vi "Execute.vi"(8 "error in (no error)":errorcluster, 9 "Workspace":T1, 10 "Cluster":T2={"I-O.lvclass"=refnum, "Gantry"=refnum, "Dispenser"="COM1"}, 11 "Pick and Place in":refnum<class "Pick and Place.lvclass">) -> (0 "error out":errorcluster, 2 "Control Out":T2={"I-O.lvclass"=refnum, "Gantry"=refnum, "Dispenser"="COM1"}, 3 "Pick and Place out":refnum<class "Pick and Place.lvclass">)   [LabVIEW 2021, in "Pick and Place.lvclass"]
uses:
  Pick and Place.lvclass
  Controller/Controllers.ctl
  Controller/I-O/I-O.lvclass
  C:/Program Files (x86)/Aerotech/A3200/LabVIEW/2010/Bin/Aerotech.A3200.dll
  Program Files (x86)/Aerotech/A3200/LabVIEW/2010/Bin/Aerotech.A3200.dll
  Workspace/Workspace.ctl
  Pick and Place Type.ctl
  Pick and Place.lvclass/Pick and Place.ctl
  4c518ff3-1de9-431e-b450-1fb7357d944a.vi
  Drivers/Aerotech A3200/Parameters/GetAxisParameterDouble.vi
  Controller/Motion/Motion.lvclass
  Drivers/Aerotech A3200/Aerotech.lvlib
  Controller/Motion/A3200/A3200.lvclass
  Controller/Controller.lvclass
  Workspace/Fixture.lvclass
panel:
  in  "Deactivate curtain?":bool
  out "Seconary Pickup time 2":timestamp
  out "Seconary Pickup time 1":timestamp
  out "milliseconds to wait":u32
  out "XYZTheta Out":dbl[](array[numeric])
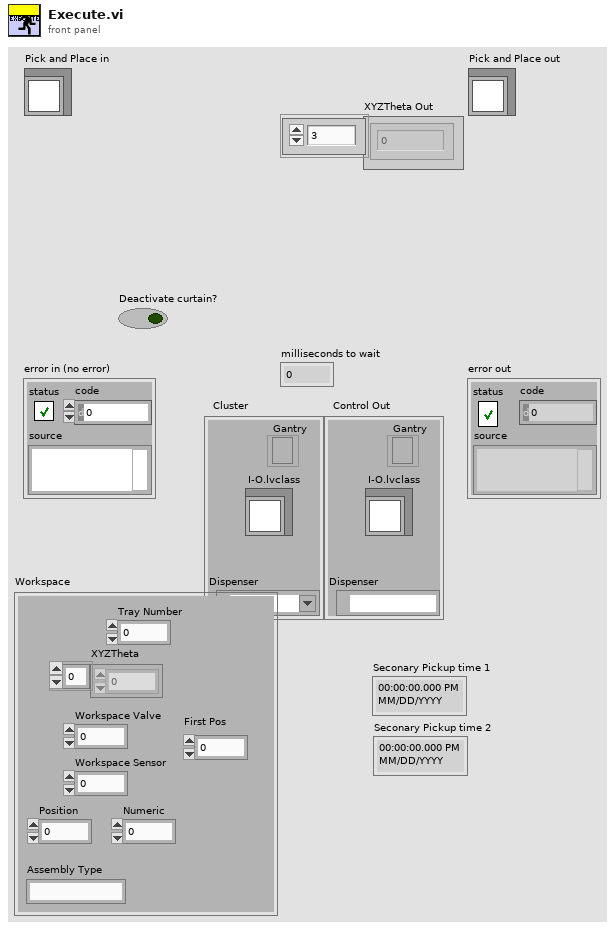
[diagram p1: front panel]
types:
  T1 = typedef "Fixture.lvclass/Workspace.ctl" = cluster{"XYZTheta":dbl[], "Workspace Valve":i32, "Workspace Sensor":i32, "Tray Number":i32, "Position":i32, "Assembly Type":string, "Numeric":dbl, "First Pos":i32}
  T2 = typedef "Controller.lvclass/Controllers.ctl" = cluster{"I-O.lvclass":refnum<class "I-O.lvclass">, "Gantry":refnum<k24>, "Dispenser":refnum<visa-resource-name>}
  T3 = typedef "Pick and Place.lvclass/Pick and Place Type.ctl" = enum16{"Primary Pick Up", "Secondary Pick Up", "Put Down All", "Pick Up All", "Put Down Secondary"}
  T4 = typedef "I-O.lvclass/Pin Map.ctl" = cluster{"Region Valves":i32[], "Extra Valves":dbl[][][], "Tool Primary Valve":i32, "Tool Secondary Valve":i32, "Region Sensors":i32[], "Extra Sensors":dbl[][][], "Tool Primary Sensor":dbl, "Tool Secondary Sensor":dbl, "Compression Sensor":dbl, "5V":i32, "Dispenser Sensor":dbl, "Light Curtain":i32}
  T5 = cluster{"Status":bool, "Error Code":i32, "Source":string}
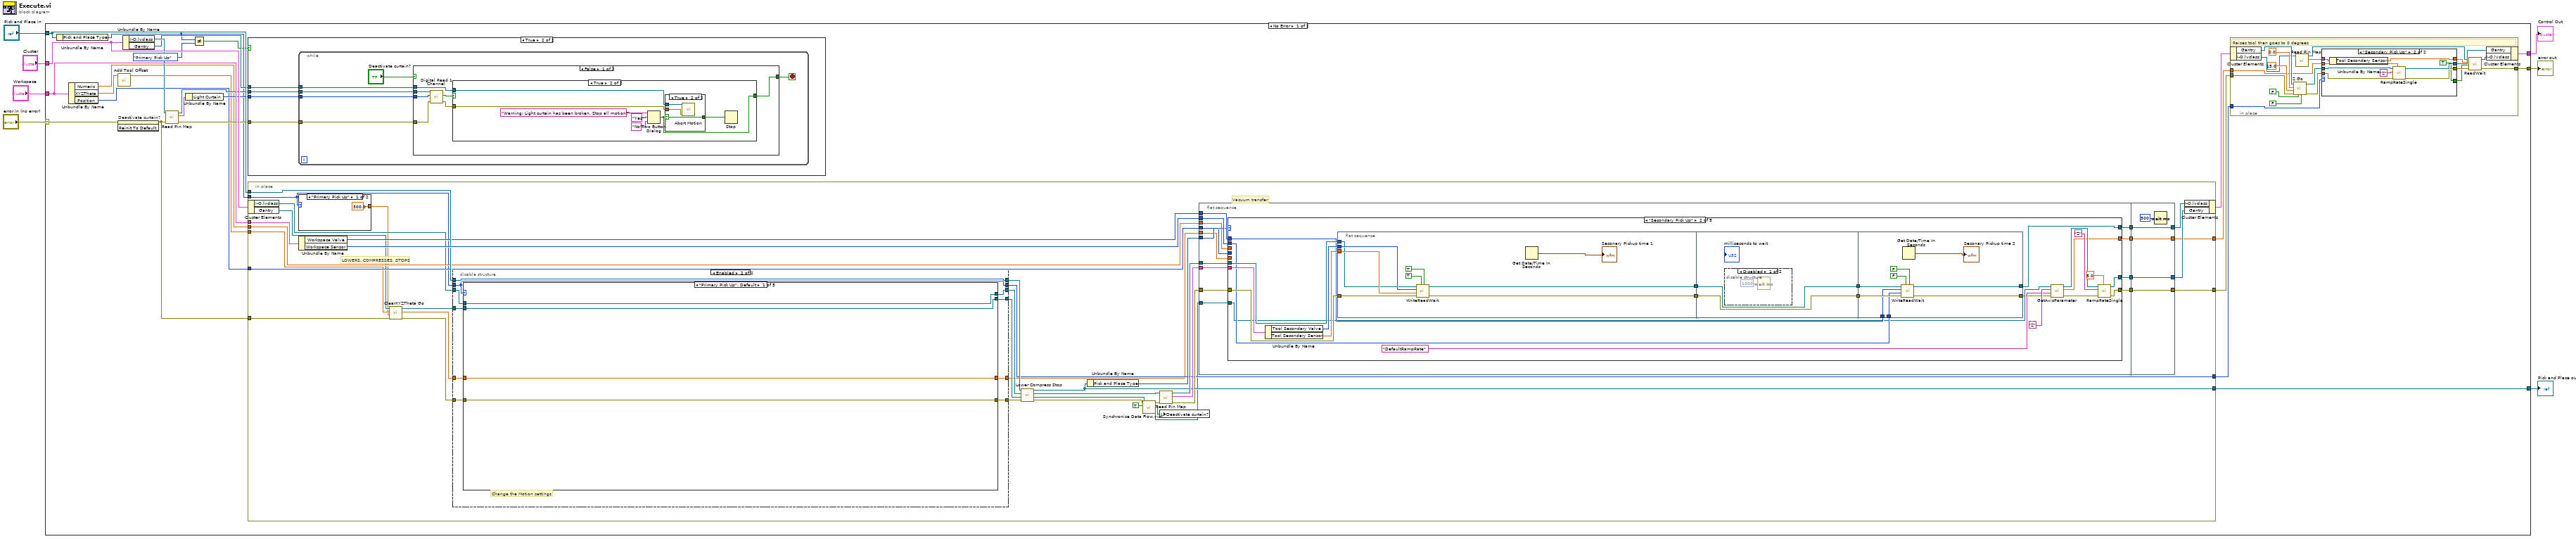
[diagram p0: block diagram]
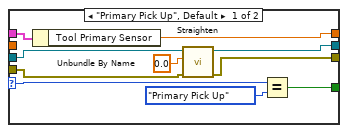
[diagram p6: hidden frame]
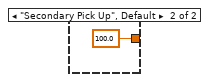
[diagram p7: hidden frame]
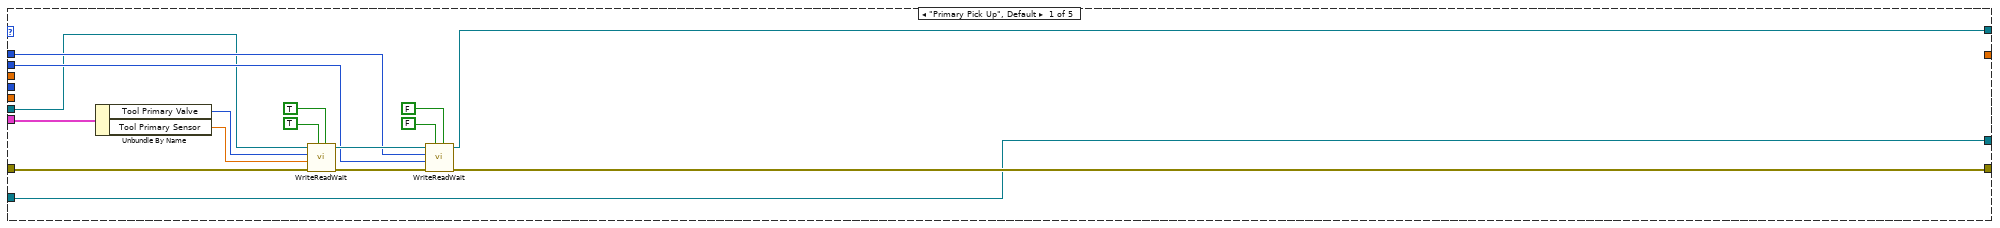
[diagram p8: hidden frame]
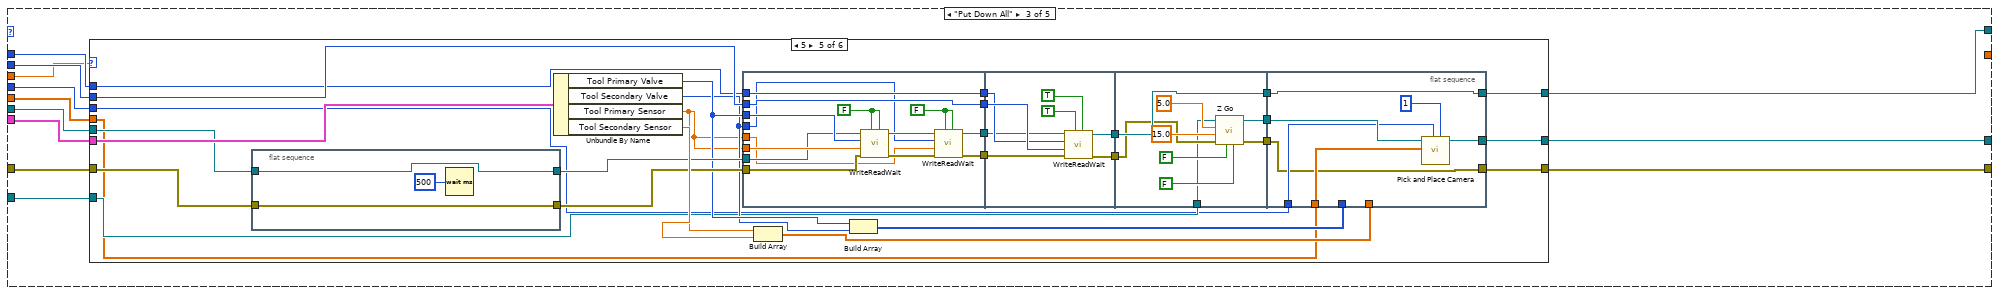
[diagram p10: hidden frame]
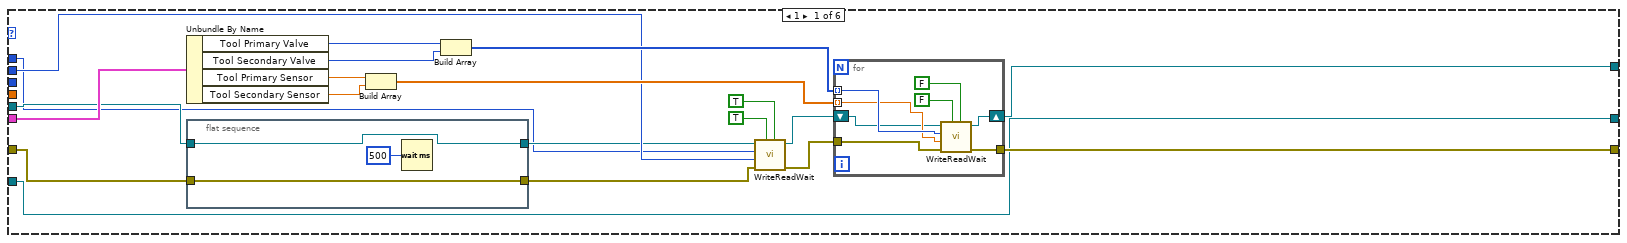
[diagram p11: hidden frame]
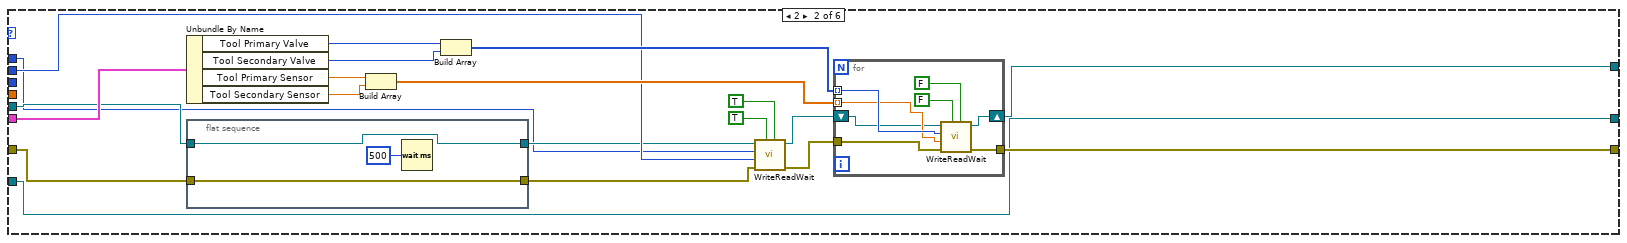
[diagram p12: hidden frame]
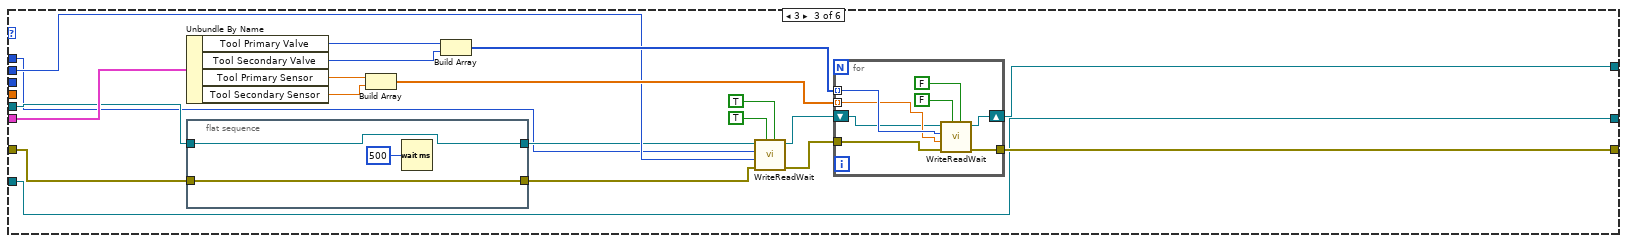
[diagram p13: hidden frame]
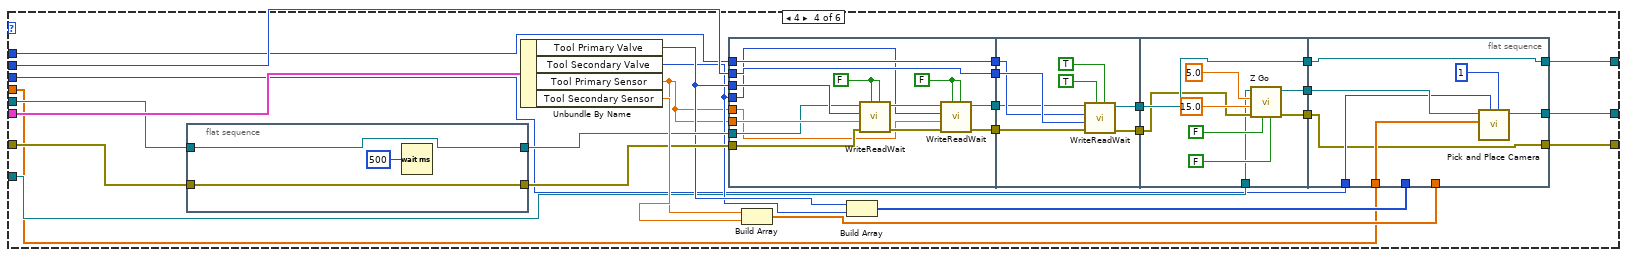
[diagram p14: hidden frame]
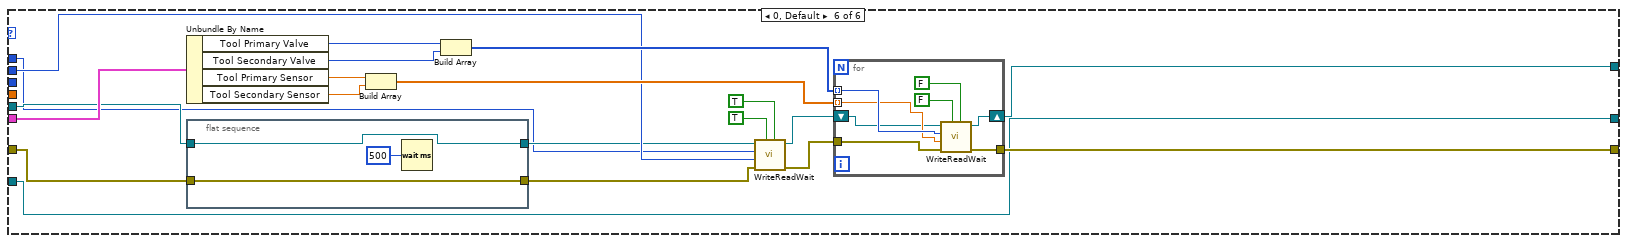
[diagram p15: hidden frame]
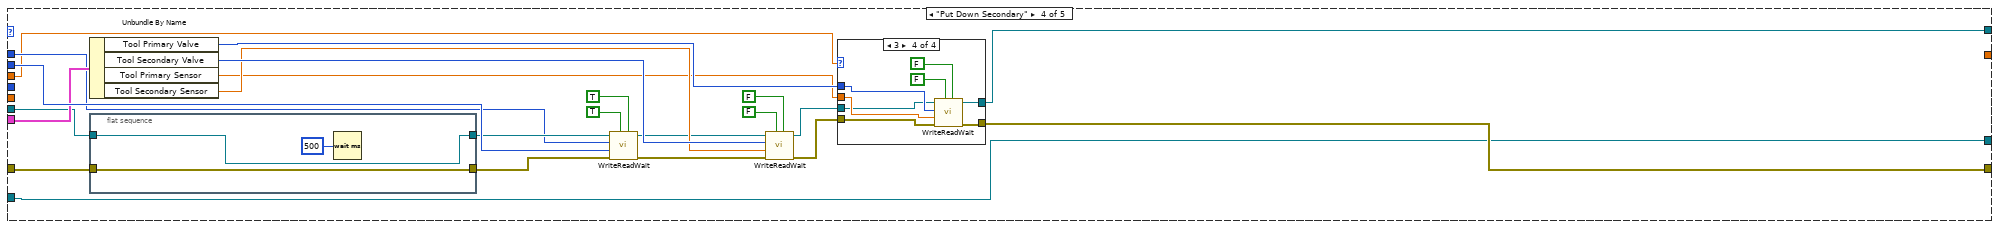
[diagram p16: hidden frame]
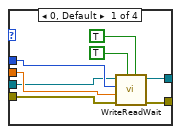
[diagram p17: hidden frame]
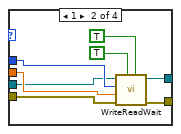
[diagram p18: hidden frame]
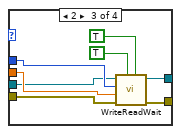
[diagram p19: hidden frame]
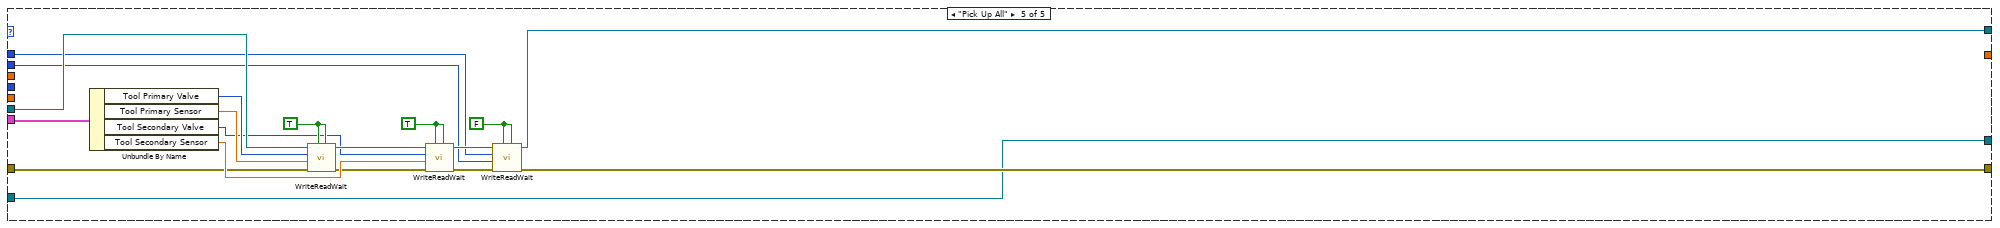
[diagram p20: hidden frame]
diagram:
  n1 = case shown="No Error" "error in (no error)" {
    selector: "error in (no error)" -> [w16 w646]
    tunnel: "Cluster" -> [w22 w647]
    tunnel: "Workspace" -> [w32 _]
    tunnel: [w29 w646] -> w1
    tunnel: [w31 w647] -> w2
    tunnel: "Pick and Place in" -> [w26 w645]
    tunnel: [w30 w645] -> w6
    frame No Error {
      n2 = Unbundle By Name(w26) -> ("Pick and Place Type"=w12:T3)
      n3 = Unbundle By Name(w32) -> ("Numeric"=w8:dbl, "XYZTheta"=w24:dbl[], "Position"=w9:i32)
      n4 = call "Add Tool Offset.vi"("XYZTheta"=w24) -> ("Array"=w13:dbl[])  [unwired: 10 in]
      n5 = invoke on="Deactivate curtain?" class="Bool (strict)" method="Reinit To Default"(error in=w16) -> (error out=w14:errorcluster)  [unwired: 2 in, 2 out]
      n6 = Unbundle By Name(w22) -> ("I-O.lvclass"=w21:refnum<class "I-O.lvclass">, "Gantry"=w15:refnum<k24>)
      n7 = call-dynamic "Read Pin Map.vi"("error in (no error)"=w14, "I-O in"=w21) -> ("error out"=w19:errorcluster, "Pin Map 2"=w20:T4, "I-O out"=w18:refnum<class "I-O.lvclass">)  [unwired: 7 in]
      n8 = Unbundle By Name(w20) -> ("Light Curtain"=w17:i32)
      n9 = Not Equal?(x=w12, y=Pick_and_Place_Type."Primary Pick Up") -> (x != y?=w10:bool)
      n10 = case shown="True" w10 {
        tunnel: w19 -> [_ w36]
        tunnel: w18 -> [_ w35]
        tunnel: w17 -> [_ w34]
        tunnel: w15 -> [_ w33]
        frame False {
        }
        frame True {
          n11 = while {
            tunnel: w36 -> [w40]
            tunnel: w35 -> [w39]
            tunnel: w34 -> [w38]
            tunnel: w33 -> [w37]
            stop <- w42 stop-if-true
            n12 = case shown="False" "Deactivate curtain?" {
              selector: "Deactivate curtain?" -> [_ w62]
              tunnel: w38 -> [w49 _]
              tunnel: w39 -> [w48 _]
              tunnel: w40 -> [w47 _]
              tunnel: [w45 w62] -> w42
              tunnel: w37 -> [w44 _]
              frame False {
                n13 = call-dynamic "Digital Read 1 Channel.vi"("error in (no error)"=w47, "Read"=w49, "I-O in"=w48) -> ("error out"=w43:errorcluster, "Value"=w46:bool)  [unwired: 6 in, 1 out]
                n14 = case shown="True" w46 {
                  selector: w46 -> [w50 _]
                  tunnel: [w50 w54] -> w45
                  tunnel: w44 -> [_ w53]
                  tunnel: w43 -> [_ w52]
                  frame False {
                  }
                  frame True {
                    n15 = Two Button Dialog(message="Warning: Light curtain has been broken. Stop all motion?", 1:"No" ("F button name (\"Cancel\")"), 2:"Yes" ("T button name (\"OK\")")) -> (T button?=w54:bool)
                    n16 = case shown="True" w54 {
                      selector: w54 -> [w58 w59]
                      tunnel: w53 -> [_ w61]
                      tunnel: w52 -> [_ w60]
                      tunnel: [w58 w59] -> w51
                      frame False {
                      }
                      frame True {
                        n17 = call "Abort Motion.vi"("error in (no error)"=w60, "Gantry In"=w61) -> ()  [unwired: 8 in, 2 out]
                      }
                    }
                    n18 = Stop(stop? (T)=w51) -> ()
                  }
                }
              }
              frame True {
              }
            }
          }
        }
      }
      n19 = in-place {
        in-place-border: w32 -> [w141]
        in-place-border: w26 -> [w131]
        in-place-border: [w135] -> w30
        in-place-border: [w133] -> w27
        in-place-border: w12 -> [w102]
        in-place-border: [w125] -> w25
        in-place-border: w8 -> [w124]
        in-place-border: w9 -> [w121]
        in-place-border: [w120] -> w23
        in-place-border: w14 -> [w108]
        in-place-border: w13 -> [w107]
        # "Vacuum transfer"
        # "LOWERS, COMPRESSES, STOPS"
        n20 = in-place-cluster #1(w22) -> ("I-O.lvclass"=w115:refnum<class "I-O.lvclass">, "Gantry"=w104:refnum<k24>)
        n21 = case shown="\"Primary Pick Up\"" w102 {
          tunnel: [300.0 ("Speed") 100.0 ("Speed")] -> w101
          frame "Primary Pick Up" {
          }
          frame "Secondary Pick Up", Default {
          }
        }
        n22 = Unbundle By Name(w141) -> ("Workspace Valve"=w128:i32, "Workspace Sensor"=w140:i32)
        n23 = call "ClearXYZTheta Go.vi"("error in (no error)"=w108, "Speed"=w101, "XYZTheta In"=w107, "Gantry In"=w104) -> ("error out"=w106:errorcluster, "XYZTheta Out"=w105:dbl[], "Gantry Out"=w103:refnum<k24>)  [unwired: 5 in]
        n24 = disable-structure shown="Enabled" {
          disable-tunnel: [w578 w588] -> w132
          disable-tunnel: w131 -> [w578 w588]
          disable-tunnel: w115 -> [w577 w587]
          disable-tunnel: [w577 w586] -> w130
          disable-tunnel: w103 -> [w576 w582]
          disable-tunnel: w106 -> [w575 w585]
          disable-tunnel: [w575 w584] -> w129
          disable-tunnel: w102 -> [w574 w580]
          disable-tunnel: [_ w583] -> w127
          disable-tunnel: w105 -> [_ w581]
          disable-tunnel: [_ w580] -> w125
          disable-tunnel: [_ w579] -> w123
          frame Disabled {
          }
          frame Enabled {
            # "Change the Motion settings"
            n25 = case shown="\"Primary Pick Up\", Default" w580 {
              tunnel: w587 -> [w592 w596 w600 w604 w644]
              tunnel: [w592 w596 w600 w604 w644] -> w586
              tunnel: w585 -> [w591 w595 w599 w603 w636]
              tunnel: [w591 w595 w599 w603 w613] -> w584
              tunnel: [w590 w594 w598 w602 w612] -> w583
              tunnel: w582 -> [w590 w594 w598 w602 w638]
              tunnel: w581 -> [w589 w593 w597 w601 w643]
              tunnel: [w589 w593 w597 w601 w605] -> w579
              frame "Primary Pick Up", Default {
              }
              frame "Secondary Pick Up" {
              }
              frame "Put Down All" {
              }
              frame "Pick Up All" {
              }
              frame "Put Down Secondary" {
                w639 = dbl[] [0.0, 0.0, 0.0, 0.0] ("y")
                w640 = dbl[] [0.0, 0.0, 0.0, 0.0] ("y")
                w641 = dbl[] [0.0, 0.0, 0.0, 0.0] ("y")
                w642 = dbl[] [0.0, 0.0, 0.0, 0.0] ("y")
                # "at 33 mm normally"
                # "In Radians\n\npositive = Clockwise\nNegative = Counterclockwise\n\n0.174533 = 10 degrees"
                # "Theta Motion"
                # "0 is the left side\nPositive = Go Right\nNegative = Go Left"
                # "0 is the back\nPositive = Go Forward\nNegative = Go Backwards"
                # "0 is top, about 80 is the tray\npositive = Go Down\nNegative = Go Up"
                # "Z Motion"
                # "Y Motion"
                # "X Motion"
                n26 = disable-structure shown="Disabled" {
                  frame Disabled {
                    n27 = call "ClearXYZTheta Go.vi"() -> ()  [unwired: 9 in, 3 out]
                  }
                  frame Enabled {
                  }
                }
                n28 = Add(x=w643, y=w642) -> (x+y=w637:dbl[])
                n29 = call "XYZThetaGo.vi"("error in (no error)"=w636, "XYZTheta In"=w637, "Gantry In"=w638) -> ("error out"=w632:errorcluster, "XYZTheta Out"=w635:dbl[], "Gantry Out"=w634:refnum<k24>)  [unwired: 6 in]
                n30 = Subtract(x=w635, y=w642) -> (x-y=w633:dbl[])
                n31 = call "XYZThetaGo.vi"("error in (no error)"=w632, "XYZTheta In"=w633, "Gantry In"=w634) -> ("error out"=w609:errorcluster, "XYZTheta Out"=w631:dbl[], "Gantry Out"=w611:refnum<k24>)  [unwired: 6 in]
                n32 = Add(x=w631, y=w641) -> (x+y=w610:dbl[])
                n33 = call "XYZThetaGo.vi"("error in (no error)"=w609, "XYZTheta In"=w610, "Gantry In"=w611) -> ("error out"=w608:errorcluster, "XYZTheta Out"=w607:dbl[], "Gantry Out"=w606:refnum<k24>)  [unwired: 6 in]
                n34 = Subtract(x=w607, y=w641) -> (x-y=w629:dbl[])
                n35 = call "XYZThetaGo.vi"("error in (no error)"=w608, "XYZTheta In"=w629, "Gantry In"=w606) -> ("error out"=w625:errorcluster, "XYZTheta Out"=w630:dbl[], "Gantry Out"=w628:refnum<k24>)  [unwired: 6 in]
                n36 = Add(x=w630, y=w640) -> (x+y=w626:dbl[])
                n37 = call "XYZThetaGo.vi"("error in (no error)"=w625, "XYZTheta In"=w626, "Gantry In"=w628) -> ("error out"=w622:errorcluster, "XYZTheta Out"=w627:dbl[], "Gantry Out"=w624:refnum<k24>)  [unwired: 6 in]
                n38 = Subtract(x=w627, y=w640) -> (x-y=w623:dbl[])
                n39 = call "XYZThetaGo.vi"("error in (no error)"=w622, "XYZTheta In"=w623, "Gantry In"=w624) -> ("error out"=w618:errorcluster, "XYZTheta Out"=w621:dbl[], "Gantry Out"=w620:refnum<k24>)  [unwired: 6 in]
                n40 = Add(x=w621, y=w639) -> (x+y=w619:dbl[])
                n41 = call "XYZThetaGo.vi"("error in (no error)"=w618, "XYZTheta In"=w619, "Gantry In"=w620) -> ("error out"=w614:errorcluster, "XYZTheta Out"=w617:dbl[], "Gantry Out"=w616:refnum<k24>)  [unwired: 6 in]
                n42 = Subtract(x=w617, y=w639) -> (x-y=w615:dbl[])
                n43 = call "XYZThetaGo.vi"("error in (no error)"=w614, "XYZTheta In"=w615, "Gantry In"=w616) -> ("error out"=w613:errorcluster, "XYZTheta Out"=w605:dbl[], "Gantry Out"=w612:refnum<k24>)  [unwired: 6 in]
                "XYZTheta Out" <- w605
              }
            }
          }
        }
        n44 = call "Lower Compress Stop.vi"("error in (no error)"=w129, "Gantry In"=w127, "I-O.lvclass"=w130, "Pick and Place in"=w132) -> ("error out"=w114:errorcluster, "Gantry Out"=w110:refnum<k24>, "I-O out"=w136:refnum<class "I-O.lvclass">, "Pick and Place Out"=w135:refnum<class "Pick and Place.lvclass">)  [unwired: 4 in]
        n45 = Unbundle By Name(w135) -> ("Pick and Place Type"=w126:T3)
        n46 = call "Synchronize Data Flow.vim"("input 3"=w110, "input 2"=TRUE ("Deactivate curtain?"), "input 1"=w114) -> ("output 3"=w109:refnum<k24>, "output 2"=w112:bool, "output 1"=w113:errorcluster)  [unwired: 1 in, 1 out]
        n47 = call-dynamic "Read Pin Map.vi"("error in (no error)"=w113, "I-O in"=w136) -> ("error out"=w134:errorcluster, "Pin Map 2"=w139:T4, "I-O out"=w138:refnum<class "I-O.lvclass">)  [unwired: 7 in]
        n48 = local write "Deactivate curtain?"(w112) -> ()
        n49 = flat-sequence {
          tunnel: w140 -> [w157]
          tunnel: w139 -> [w156]
          tunnel: w138 -> [w155]
          tunnel: w134 -> [w153]
          tunnel: w128 -> [w151]
          tunnel: w126 -> [w150]
          tunnel: w124 -> [w149]
          tunnel: w123 -> [w148]
          tunnel: w109 -> [w147]
          tunnel: w121 -> [w145]
          tunnel: [w154] -> w119
          tunnel: [w152] -> w118
          tunnel: [w146] -> w117
          tunnel: [w144] -> w116
          tunnel: [w570] -> w120
          tunnel: [w571] -> w122
          tunnel: [w572] -> w133
          tunnel: [w573] -> w137
          tunnel: w119 -> [w573]
          tunnel: w118 -> [w572]
          tunnel: w117 -> [w571]
          tunnel: w116 -> [w570]
          frame #0 {
            n50 = case shown="\"Secondary Pick Up\"" w150 {
              tunnel: w151 -> [w171 w186 w223 w504 w558]
              tunnel: w157 -> [w170 w187 w228 w511 w557]
              tunnel: [w165 w185 w229 w514 w555] -> w154
              tunnel: w155 -> [w164 w194 w226 w508 w567]
              tunnel: w156 -> [w163 w193 w227 w510 w568]
              tunnel: w153 -> [w161 w192 w225 w506 w554]
              tunnel: [w159 w182 w224 w505 w551] -> w152
              tunnel: w149 -> [_ _ w218 w493 _]
              tunnel: w148 -> [_ _ w222 _ _]
              tunnel: w147 -> [w158 w178 w221 w492 w550]
              tunnel: [w158 w184 w220 w492 w550] -> w146
              tunnel: w145 -> [_ _ w219 _ _]
              tunnel: [_ w174 _ _ _] -> w144
              frame "Primary Pick Up", Default {
                n51 = Unbundle By Name(w163) -> ("Tool Primary Valve"=w162:i32, "Tool Primary Sensor"=w173:dbl)
                n52 = call "WriteReadWait.vi"("Read Value"=TRUE, "Write Value"=TRUE, "error in (no error)"=w161, "Read"=w173, "Write"=w162, "I-O in"=w164) -> ("error out"=w160:errorcluster, "I-O out"=w172:refnum<class "I-O.lvclass">)  [unwired: 4 in]
                n53 = call "WriteReadWait.vi"("Read Value"=FALSE ("Write Value"), "Write Value"=FALSE ("Read Value"), "error in (no error)"=w160, "Read"=w170, "Write"=w171, "I-O in"=w172) -> ("error out"=w159:errorcluster, "I-O out"=w165:refnum<class "I-O.lvclass">)  [unwired: 4 in]
              }
              frame "Secondary Pick Up" {
                n54 = Unbundle By Name(w193) -> ("Tool Secondary Valve"=w196:i32, "Tool Secondary Sensor"=w195:dbl)
                n55 = flat-sequence {
                  tunnel: w196 -> [w202]
                  tunnel: w195 -> [w201]
                  tunnel: w194 -> [w200]
                  tunnel: w192 -> [w199]
                  tunnel: [w205] -> w191
                  tunnel: [w198] -> w190
                  tunnel: w191 -> [w207]
                  tunnel: w190 -> [w206]
                  tunnel: [w207] -> w189
                  tunnel: [w206] -> w188
                  tunnel: w189 -> [w214]
                  tunnel: w188 -> [w217]
                  tunnel: w187 -> [w216]
                  tunnel: w186 -> [w215]
                  tunnel: [w213] -> w176
                  tunnel: [w212] -> w185
                  frame #0 {
                    n56 = call "WriteReadWait.vi"("Read Value"=TRUE, "Write Value"=TRUE, "error in (no error)"=w199, "Read"=w201, "Write"=w202, "I-O in"=w200) -> ("error out"=w198:errorcluster, "I-O out"=w205:refnum<class "I-O.lvclass">)  [unwired: 4 in]
                    n57 = Get Date/Time In Seconds() -> (seconds since 1Jan1904=→"Seconary Pickup time 1":timestamp)
                  }
                  frame #1 {
                    n58 = disable-structure shown="Disabled" {
                      frame Disabled {
                        n59 = Wait (ms)(milliseconds to wait=u32 1000) -> ()  [unwired: 1 out]
                      }
                      frame Enabled {
                      }
                    }
                  }
                  frame #2 {
                    n60 = call "WriteReadWait.vi"("Read Value"=FALSE ("Write Value"), "Write Value"=FALSE ("Read Value"), "error in (no error)"=w217, "Read"=w216, "Write"=w215, "I-O in"=w214) -> ("error out"=w213:errorcluster, "I-O out"=w212:refnum<class "I-O.lvclass">)  [unwired: 4 in]
                    n61 = Get Date/Time In Seconds() -> (seconds since 1Jan1904=→"Seconary Pickup time 2":timestamp)
                  }
                }
                n62 = call-poly "GetAxisParameter.vi"("error in (no error)"=w176, "Parameter Name"="DefaultRampRate", "axis name"="Z", "controller in"=w178) -> ("error out"=w175:errorcluster, "value"=w174:dbl, "controller out"=w177:refnum<k24>)  [unwired: 5 in]
                n63 = call "RampRateSingle.vi"("ramp rate"=5.0, "error in (no error)"=w175, "axis name"="Z", "controller in"=w177) -> ("error out (no error)"=w182:T5, "controller out"=w184:refnum<k24>)  [unwired: 6 in]
              }
              frame "Put Down All" {
                n64 = case shown="5" w218 {
                  tunnel: [w243 w274 w305 w340 w409 w474] -> w229
                  tunnel: w228 -> [w240 w271 w302 w349 w418 w471]
                  tunnel: w227 -> [w239 w270 w301 w348 w417 w470]
                  tunnel: w226 -> [w236 w267 w298 w346 w415 w467]
                  tunnel: w225 -> [w233 w264 w295 w344 w413 w464]
                  tunnel: [w232 w263 w294 w339 w408 w463] -> w224
                  tunnel: w223 -> [w231 w262 w293 w343 w412 w462]
                  tunnel: w222 -> [_ _ _ w330 w399 _]
                  tunnel: w221 -> [w230 w261 w292 w335 w404 w461]
                  tunnel: [w230 w261 w292 w331 w400 w461] -> w220
                  tunnel: w219 -> [_ _ _ w329 w398 _]
                  frame 1 {
                    n65 = Unbundle By Name(w239) -> ("Tool Primary Valve"=w244:i32, "Tool Secondary Valve"=w245:i32, "Tool Primary Sensor"=w246:dbl, "Tool Secondary Sensor"=w247:dbl)
                    n66 = flat-sequence {
                      tunnel: [w251] -> w237
                      tunnel: w236 -> [w251]
                      tunnel: [w250] -> w234
                      tunnel: w233 -> [w250]
                      frame #0 {
                        # "Delay After Placing"
                        n67 = Wait (ms)(milliseconds to wait=u32 500) -> ()  [unwired: 1 out]
                      }
                    }
                    n68 = Build Array(w246, w247) -> (w249:dbl[])
                    n69 = Build Array(w244, w245) -> (w248:i32[])
                    n70 = call "WriteReadWait.vi"("Read Value"=TRUE, "Write Value"=TRUE, "error in (no error)"=w234, "Read"=w240, "Write"=w231, "I-O in"=w237) -> ("error out"=w235:errorcluster, "I-O out"=w238:refnum<class "I-O.lvclass">)  [unwired: 4 in]
                    n71 = for {
                      shift-right: [w255] -> w243
                      shift-left: w238 -> [w256]
                      tunnel: w248 -> [w258] mode=indexing
                      tunnel: w249 -> [w257] mode=indexing
                      tunnel: w235 -> [w254]
                      tunnel: [w253] -> w232
                      n72 = call "WriteReadWait.vi"("Read Value"=FALSE ("Write Value"), "Write Value"=FALSE ("Read Value"), "error in (no error)"=w254, "Read"=w257, "Write"=w258, "I-O in"=w256) -> ("error out"=w253:errorcluster, "I-O out"=w255:refnum<class "I-O.lvclass">)  [unwired: 4 in]
                    }
                  }
                  frame 2 {
                    n73 = Unbundle By Name(w270) -> ("Tool Primary Valve"=w275:i32, "Tool Secondary Valve"=w276:i32, "Tool Primary Sensor"=w277:dbl, "Tool Secondary Sensor"=w278:dbl)
                    n74 = flat-sequence {
                      tunnel: [w282] -> w268
                      tunnel: w267 -> [w282]
                      tunnel: [w281] -> w265
                      tunnel: w264 -> [w281]
                      frame #0 {
                        # "Delay After Placing"
                        n75 = Wait (ms)(milliseconds to wait=u32 500) -> ()  [unwired: 1 out]
                      }
                    }
                    n76 = Build Array(w277, w278) -> (w280:dbl[])
                    n77 = Build Array(w275, w276) -> (w279:i32[])
                    n78 = call "WriteReadWait.vi"("Read Value"=TRUE, "Write Value"=TRUE, "error in (no error)"=w265, "Read"=w271, "Write"=w262, "I-O in"=w268) -> ("error out"=w266:errorcluster, "I-O out"=w269:refnum<class "I-O.lvclass">)  [unwired: 4 in]
                    n79 = for {
                      shift-right: [w286] -> w274
                      shift-left: w269 -> [w287]
                      tunnel: w279 -> [w289] mode=indexing
                      tunnel: w280 -> [w288] mode=indexing
                      tunnel: w266 -> [w285]
                      tunnel: [w284] -> w263
                      n80 = call "WriteReadWait.vi"("Read Value"=FALSE ("Write Value"), "Write Value"=FALSE ("Read Value"), "error in (no error)"=w285, "Read"=w288, "Write"=w289, "I-O in"=w287) -> ("error out"=w284:errorcluster, "I-O out"=w286:refnum<class "I-O.lvclass">)  [unwired: 4 in]
                    }
                  }
                  frame 3 {
                    n81 = Unbundle By Name(w301) -> ("Tool Primary Valve"=w306:i32, "Tool Secondary Valve"=w307:i32, "Tool Primary Sensor"=w308:dbl, "Tool Secondary Sensor"=w309:dbl)
                    n82 = flat-sequence {
                      tunnel: [w313] -> w299
                      tunnel: w298 -> [w313]
                      tunnel: [w312] -> w296
                      tunnel: w295 -> [w312]
                      frame #0 {
                        # "Delay After Placing"
                        n83 = Wait (ms)(milliseconds to wait=u32 500) -> ()  [unwired: 1 out]
                      }
                    }
                    n84 = Build Array(w308, w309) -> (w311:dbl[])
                    n85 = Build Array(w306, w307) -> (w310:i32[])
                    n86 = call "WriteReadWait.vi"("Read Value"=TRUE, "Write Value"=TRUE, "error in (no error)"=w296, "Read"=w302, "Write"=w293, "I-O in"=w299) -> ("error out"=w297:errorcluster, "I-O out"=w300:refnum<class "I-O.lvclass">)  [unwired: 4 in]
                    n87 = for {
                      shift-right: [w317] -> w305
                      shift-left: w300 -> [w318]
                      tunnel: w310 -> [w320] mode=indexing
                      tunnel: w311 -> [w319] mode=indexing
                      tunnel: w297 -> [w316]
                      tunnel: [w315] -> w294
                      n88 = call "WriteReadWait.vi"("Read Value"=FALSE ("Write Value"), "Write Value"=FALSE ("Read Value"), "error in (no error)"=w316, "Read"=w319, "Write"=w320, "I-O in"=w318) -> ("error out"=w315:errorcluster, "I-O out"=w317:refnum<class "I-O.lvclass">)  [unwired: 4 in]
                    }
                  }
                  frame 4 {
                    n89 = flat-sequence {
                      tunnel: [w390] -> w347
                      tunnel: w346 -> [w390]
                      tunnel: [w389] -> w345
                      tunnel: w344 -> [w389]
                      frame #0 {
                        # "Delay After Placing"
                        n90 = Wait (ms)(milliseconds to wait=u32 500) -> ()  [unwired: 1 out]
                      }
                    }
                    n91 = Unbundle By Name(w348) -> ("Tool Primary Valve"=w338:i32, "Tool Secondary Valve"=w337:i32, "Tool Primary Sensor"=w336:dbl, "Tool Secondary Sensor"=w350:dbl)
                    n92 = flat-sequence {
                      tunnel: w343 -> [w363]
                      tunnel: w345 -> [w357]
                      tunnel: w347 -> [w360]
                      tunnel: w349 -> [w364]
                      tunnel: [w364] -> w328
                      tunnel: [w358] -> w327
                      tunnel: [w355] -> w325
                      tunnel: [w363] -> w323
                      tunnel: w338 -> [w362]
                      tunnel: w336 -> [w361]
                      tunnel: w337 -> [w354]
                      tunnel: w336 -> [w353]
                      tunnel: w328 -> [w372]
                      tunnel: w327 -> [w370]
                      tunnel: [w369] -> w326
                      tunnel: w325 -> [w366]
                      tunnel: [w365] -> w324
                      tunnel: w323 -> [w371]
                      tunnel: w326 -> [w381]
                      tunnel: [w381] -> w334
                      tunnel: w324 -> [w376]
                      tunnel: [w375] -> w333
                      tunnel: w335 -> [w374]
                      tunnel: [w373] -> w332
                      tunnel: w342 -> [_]
                      tunnel: w341 -> [_]
                      tunnel: [w382] -> w340
                      tunnel: [w383] -> w339
                      tunnel: w329 -> [w385]
                      tunnel: w330 -> [w386]
                      tunnel: [w387] -> w331
                      tunnel: w332 -> [w388]
                      tunnel: w333 -> [w383]
                      tunnel: w334 -> [w382]
                      frame #0 {
                        w352 = FALSE ("Read Value")
                        w351 = FALSE ("Read Value")
                        n93 = call "WriteReadWait.vi"("Read Value"=w352, "Write Value"=w352, "error in (no error)"=w357, "Read"=w361, "Write"=w362, "I-O in"=w360) -> ("error out"=w356:errorcluster, "I-O out"=w359:refnum<class "I-O.lvclass">)  [unwired: 4 in]
                        n94 = call "WriteReadWait.vi"("Read Value"=w351, "Write Value"=w351, "error in (no error)"=w356, "Read"=w353, "Write"=w354, "I-O in"=w359) -> ("error out"=w355:errorcluster, "I-O out"=w358:refnum<class "I-O.lvclass">)  [unwired: 4 in]
                      }
                      frame #1 {
                        n95 = call "WriteReadWait.vi"("Read Value"=TRUE, "Write Value"=TRUE ("Read Value"), "error in (no error)"=w366, "Read"=w372, "Write"=w371, "I-O in"=w370) -> ("error out"=w365:errorcluster, "I-O out"=w369:refnum<class "I-O.lvclass">)  [unwired: 4 in]
                      }
                      frame #2 {
                        n96 = call "Z Go.vi"("Increment"=FALSE, "Return Immediately"=FALSE ("Increment"), "error in (no error)"=w376, "Speed In"=15.0 ("speed"), "Position In"=5.0 ("position"), "Gantry In"=w374) -> ("error out"=w375:errorcluster, "Gantry Out"=w373:refnum<k24>)  [unwired: 2 in, 2 out]
                      }
                      frame #3 {
                        n97 = call "Pick and Place Camera.vi"("Gantry In"=w388, "XYZTheta"=w386, "Position"=w385, "Tray Number"=1) -> ("Gantry Out"=w387:refnum<k24>)  [unwired: 6 in]
                      }
                    }
                    n98 = Build Array(w336, w350) -> (w341:dbl[])
                    n99 = Build Array(w338, w337) -> (w342:i32[])
                  }
                  frame 5 {
                    n100 = flat-sequence {
                      tunnel: [w459] -> w416
                      tunnel: w415 -> [w459]
                      tunnel: [w458] -> w414
                      tunnel: w413 -> [w458]
                      frame #0 {
                        # "Delay After Placing"
                        n101 = Wait (ms)(milliseconds to wait=u32 500) -> ()  [unwired: 1 out]
                      }
                    }
                    n102 = Unbundle By Name(w417) -> ("Tool Primary Valve"=w407:i32, "Tool Secondary Valve"=w406:i32, "Tool Primary Sensor"=w405:dbl, "Tool Secondary Sensor"=w419:dbl)
                    n103 = flat-sequence {
                      tunnel: w412 -> [w432]
                      tunnel: w414 -> [w426]
                      tunnel: w416 -> [w429]
                      tunnel: w418 -> [w433]
                      tunnel: [w433] -> w397
                      tunnel: [w427] -> w396
                      tunnel: [w424] -> w394
                      tunnel: [w432] -> w392
                      tunnel: w407 -> [w431]
                      tunnel: w405 -> [w430]
                      tunnel: w406 -> [w423]
                      tunnel: w405 -> [w422]
                      tunnel: w397 -> [w441]
                      tunnel: w396 -> [w439]
                      tunnel: [w438] -> w395
                      tunnel: w394 -> [w435]
                      tunnel: [w434] -> w393
                      tunnel: w392 -> [w440]
                      tunnel: w395 -> [w450]
                      tunnel: [w450] -> w403
                      tunnel: w393 -> [w445]
                      tunnel: [w444] -> w402
                      tunnel: w404 -> [w443]
                      tunnel: [w442] -> w401
                      tunnel: w411 -> [_]
                      tunnel: w410 -> [_]
                      tunnel: [w451] -> w409
                      tunnel: [w452] -> w408
                      tunnel: w398 -> [w454]
                      tunnel: w399 -> [w455]
                      tunnel: [w456] -> w400
                      tunnel: w401 -> [w457]
                      tunnel: w402 -> [w452]
                      tunnel: w403 -> [w451]
                      frame #0 {
                        w421 = FALSE ("Read Value")
                        w420 = FALSE ("Read Value")
                        n104 = call "WriteReadWait.vi"("Read Value"=w421, "Write Value"=w421, "error in (no error)"=w426, "Read"=w430, "Write"=w431, "I-O in"=w429) -> ("error out"=w425:errorcluster, "I-O out"=w428:refnum<class "I-O.lvclass">)  [unwired: 4 in]
                        n105 = call "WriteReadWait.vi"("Read Value"=w420, "Write Value"=w420, "error in (no error)"=w425, "Read"=w422, "Write"=w423, "I-O in"=w428) -> ("error out"=w424:errorcluster, "I-O out"=w427:refnum<class "I-O.lvclass">)  [unwired: 4 in]
                      }
                      frame #1 {
                        n106 = call "WriteReadWait.vi"("Read Value"=TRUE, "Write Value"=TRUE ("Read Value"), "error in (no error)"=w435, "Read"=w441, "Write"=w440, "I-O in"=w439) -> ("error out"=w434:errorcluster, "I-O out"=w438:refnum<class "I-O.lvclass">)  [unwired: 4 in]
                      }
                      frame #2 {
                        n107 = call "Z Go.vi"("Increment"=FALSE, "Return Immediately"=FALSE ("Increment"), "error in (no error)"=w445, "Speed In"=15.0 ("speed"), "Position In"=5.0 ("position"), "Gantry In"=w443) -> ("error out"=w444:errorcluster, "Gantry Out"=w442:refnum<k24>)  [unwired: 2 in, 2 out]
                      }
                      frame #3 {
                        n108 = call "Pick and Place Camera.vi"("Gantry In"=w457, "XYZTheta"=w455, "Position"=w454, "Tray Number"=1) -> ("Gantry Out"=w456:refnum<k24>)  [unwired: 6 in]
                      }
                    }
                    n109 = Build Array(w405, w419) -> (w410:dbl[])
                    n110 = Build Array(w407, w406) -> (w411:i32[])
                  }
                  frame 0, Default {
                    n111 = Unbundle By Name(w470) -> ("Tool Primary Valve"=w475:i32, "Tool Secondary Valve"=w476:i32, "Tool Primary Sensor"=w477:dbl, "Tool Secondary Sensor"=w478:dbl)
                    n112 = flat-sequence {
                      tunnel: [w482] -> w468
                      tunnel: w467 -> [w482]
                      tunnel: [w481] -> w465
                      tunnel: w464 -> [w481]
                      frame #0 {
                        # "Delay After Placing"
                        n113 = Wait (ms)(milliseconds to wait=u32 500) -> ()  [unwired: 1 out]
                      }
                    }
                    n114 = Build Array(w477, w478) -> (w480:dbl[])
                    n115 = Build Array(w475, w476) -> (w479:i32[])
                    n116 = call "WriteReadWait.vi"("Read Value"=TRUE, "Write Value"=TRUE, "error in (no error)"=w465, "Read"=w471, "Write"=w462, "I-O in"=w468) -> ("error out"=w466:errorcluster, "I-O out"=w469:refnum<class "I-O.lvclass">)  [unwired: 4 in]
                    n117 = for {
                      shift-right: [w486] -> w474
                      shift-left: w469 -> [w487]
                      tunnel: w479 -> [w489] mode=indexing
                      tunnel: w480 -> [w488] mode=indexing
                      tunnel: w466 -> [w485]
                      tunnel: [w484] -> w463
                      n118 = call "WriteReadWait.vi"("Read Value"=FALSE ("Write Value"), "Write Value"=FALSE ("Read Value"), "error in (no error)"=w485, "Read"=w488, "Write"=w489, "I-O in"=w487) -> ("error out"=w484:errorcluster, "I-O out"=w486:refnum<class "I-O.lvclass">)  [unwired: 4 in]
                    }
                  }
                }
              }
              frame "Put Down Secondary" {
                n119 = Unbundle By Name(w510) -> ("Tool Primary Valve"=w502:i32, "Tool Secondary Valve"=w503:i32, "Tool Primary Sensor"=w500:dbl, "Tool Secondary Sensor"=w501:dbl)
                n120 = flat-sequence {
                  tunnel: [w548] -> w509
                  tunnel: w508 -> [w548]
                  tunnel: [w547] -> w507
                  tunnel: w506 -> [w547]
                  frame #0 {
                    # "Delay After Placing"
                    n121 = Wait (ms)(milliseconds to wait=u32 500) -> ()  [unwired: 1 out]
                  }
                }
                n122 = call "WriteReadWait.vi"("Read Value"=TRUE, "Write Value"=TRUE, "error in (no error)"=w507, "Read"=w511, "Write"=w504, "I-O in"=w509) -> ("error out"=w494:errorcluster, "I-O out"=w495:refnum<class "I-O.lvclass">)  [unwired: 4 in]
                n123 = call "WriteReadWait.vi"("Read Value"=FALSE, "Write Value"=FALSE ("Read Value"), "error in (no error)"=w494, "Read"=w501, "Write"=w503, "I-O in"=w495) -> ("error out"=w496:errorcluster, "I-O out"=w497:refnum<class "I-O.lvclass">)  [unwired: 4 in]
                n124 = case shown="3" w493 {
                  tunnel: [w522 w530 w538 w546] -> w514
                  tunnel: [w521 w529 w537 w545] -> w505
                  tunnel: w502 -> [w520 w528 w536 w544]
                  tunnel: w500 -> [w519 w527 w535 w543]
                  tunnel: w497 -> [w518 w526 w534 w542]
                  tunnel: w496 -> [w515 w523 w531 w539]
                  frame 0, Default {
                    n125 = call "WriteReadWait.vi"("Read Value"=TRUE, "Write Value"=TRUE ("Read Value"), "error in (no error)"=w515, "Read"=w519, "Write"=w520, "I-O in"=w518) -> ("error out"=w521:errorcluster, "I-O out"=w522:refnum<class "I-O.lvclass">)  [unwired: 4 in]
                  }
                  frame 1 {
                    n126 = call "WriteReadWait.vi"("Read Value"=TRUE, "Write Value"=TRUE ("Read Value"), "error in (no error)"=w523, "Read"=w527, "Write"=w528, "I-O in"=w526) -> ("error out"=w529:errorcluster, "I-O out"=w530:refnum<class "I-O.lvclass">)  [unwired: 4 in]
                  }
                  frame 2 {
                    n127 = call "WriteReadWait.vi"("Read Value"=TRUE, "Write Value"=TRUE ("Read Value"), "error in (no error)"=w531, "Read"=w535, "Write"=w536, "I-O in"=w534) -> ("error out"=w537:errorcluster, "I-O out"=w538:refnum<class "I-O.lvclass">)  [unwired: 4 in]
                  }
                  frame 3 {
                    n128 = call "WriteReadWait.vi"("Read Value"=FALSE, "Write Value"=FALSE ("Read Value"), "error in (no error)"=w539, "Read"=w543, "Write"=w544, "I-O in"=w542) -> ("error out"=w545:errorcluster, "I-O out"=w546:refnum<class "I-O.lvclass">)  [unwired: 4 in]
                  }
                }
              }
              frame "Pick Up All" {
                w556 = FALSE ("Read Value")
                w560 = TRUE ("Write Value")
                w566 = TRUE ("Write Value")
                n129 = Unbundle By Name(w568) -> ("Tool Primary Valve"=w565:i32, "Tool Primary Sensor"=w564:dbl, "Tool Secondary Valve"=w562:i32, "Tool Secondary Sensor"=w561:dbl)
                n130 = call "WriteReadWait.vi"("Read Value"=w566, "Write Value"=w566, "error in (no error)"=w554, "Read"=w564, "Write"=w565, "I-O in"=w567) -> ("error out"=w553:errorcluster, "I-O out"=w563:refnum<class "I-O.lvclass">)  [unwired: 4 in]
                n131 = call "WriteReadWait.vi"("Read Value"=w560, "Write Value"=w560, "error in (no error)"=w553, "Read"=w561, "Write"=w562, "I-O in"=w563) -> ("error out"=w552:errorcluster, "I-O out"=w559:refnum<class "I-O.lvclass">)  [unwired: 4 in]
                n132 = call "WriteReadWait.vi"("Read Value"=w556, "Write Value"=w556, "error in (no error)"=w552, "Read"=w557, "Write"=w558, "I-O in"=w559) -> ("error out"=w551:errorcluster, "I-O out"=w555:refnum<class "I-O.lvclass">)  [unwired: 4 in]
              }
            }
          }
          frame #1 {
            n133 = Wait (ms)(milliseconds to wait=500) -> ()  [unwired: 1 out]
          }
        }
        n134 = in-place-cluster #1("I-O.lvclass"=w137, "Gantry"=w122) -> (w28:T2)
      }
      n135 = in-place {
        in-place-border: [w67] -> w29
        in-place-border: w27 -> [w79]
        in-place-border: w25 -> [w72]
        in-place-border: w23 -> [w71]
        # "Raises tool then goes to 0 degrees"
        n136 = in-place-cluster #2(w28) -> ("Gantry"=w76:refnum<k24>, "I-O.lvclass"=w64:refnum<class "I-O.lvclass">)
        n137 = call "Z Go.vi"("Increment"=FALSE, "Return Immediately"=FALSE ("Increment"), "error in (no error)"=w79, "Speed In"=15.0 ("speed"), "Position In"=0.0 ("position"), "Gantry In"=w76) -> ("error out"=w74:errorcluster, "Gantry Out"=w78:refnum<k24>)  [unwired: 2 in, 2 out]
        n138 = call-dynamic "Read Pin Map.vi"("I-O in"=w64) -> ("Pin Map 2"=w65:T4, "I-O out"=w63:refnum<class "I-O.lvclass">)  [unwired: 8 in, 1 out]
        n139 = case shown="\"Secondary Pick Up\"" w72 {
          selector: w72 -> [w87 _]
          tunnel: w78 -> [w91 w99]
          tunnel: [w90 w98] -> w77
          tunnel: w74 -> [w89 w97]
          tunnel: w71 -> [_ w96]
          tunnel: [w85 w95] -> w70
          tunnel: [w84 TRUE] -> w69
          tunnel: [w83 w92] -> w68
          tunnel: w65 -> [w82 w93]
          frame "Primary Pick Up", Default {
            n140 = Unbundle By Name(w82) -> ("Tool Primary Sensor"=w83:dbl)
            n141 = call "Straighten.vi"("error in (no error)"=w89, "Angle (rad)"=0.0, "Gantry In"=w91) -> ("error out"=w85:errorcluster, "Gantry Out"=w90:refnum<k24>)  [unwired: 7 in]
            n142 = Equal?(x=w87, y=Pick_and_Place_Type."Primary Pick Up") -> (x = y?=w84:bool)
          }
          frame "Secondary Pick Up" {
            n143 = Unbundle By Name(w93) -> ("Tool Secondary Sensor"=w92:dbl)
            n144 = call "RampRateSingle.vi"("ramp rate"=w96, "error in (no error)"=w97, "axis name"="Z", "controller in"=w99) -> ("error out (no error)"=w95:T5, "controller out"=w98:refnum<k24>)  [unwired: 6 in]
          }
        }
        n145 = call "ReadWait.vi"("error in (no error)"=w70, "Value"=w69, "Read"=w68, "I-O in"=w63) -> ("error out"=w67:errorcluster, "I-O out"=w66:refnum<class "I-O.lvclass">)  [unwired: 6 in]
        n146 = in-place-cluster #2("Gantry"=w77, "I-O.lvclass"=w66) -> (w31:T2)
      }
    }
    frame Error {
    }
  }
  "error out" <- w1
  "Pick and Place out" <- w6
  "Control Out" <- w2
